vi "Read_Xml_Experiment.vi"(8 "error in":errorcluster) -> (0 "error out":errorcluster)   [LabVIEW 2023]
uses:
  TypeDef/Method_Info.ctl
panel:
  out "Method_Fit 2":T2
  in  "Method_Fit":T2
  in  "Method_Fit":T1[](array[typedef])
  out "Method_Fit":T1[](array[typedef])
  out "text":string
  in  "Xml path":path
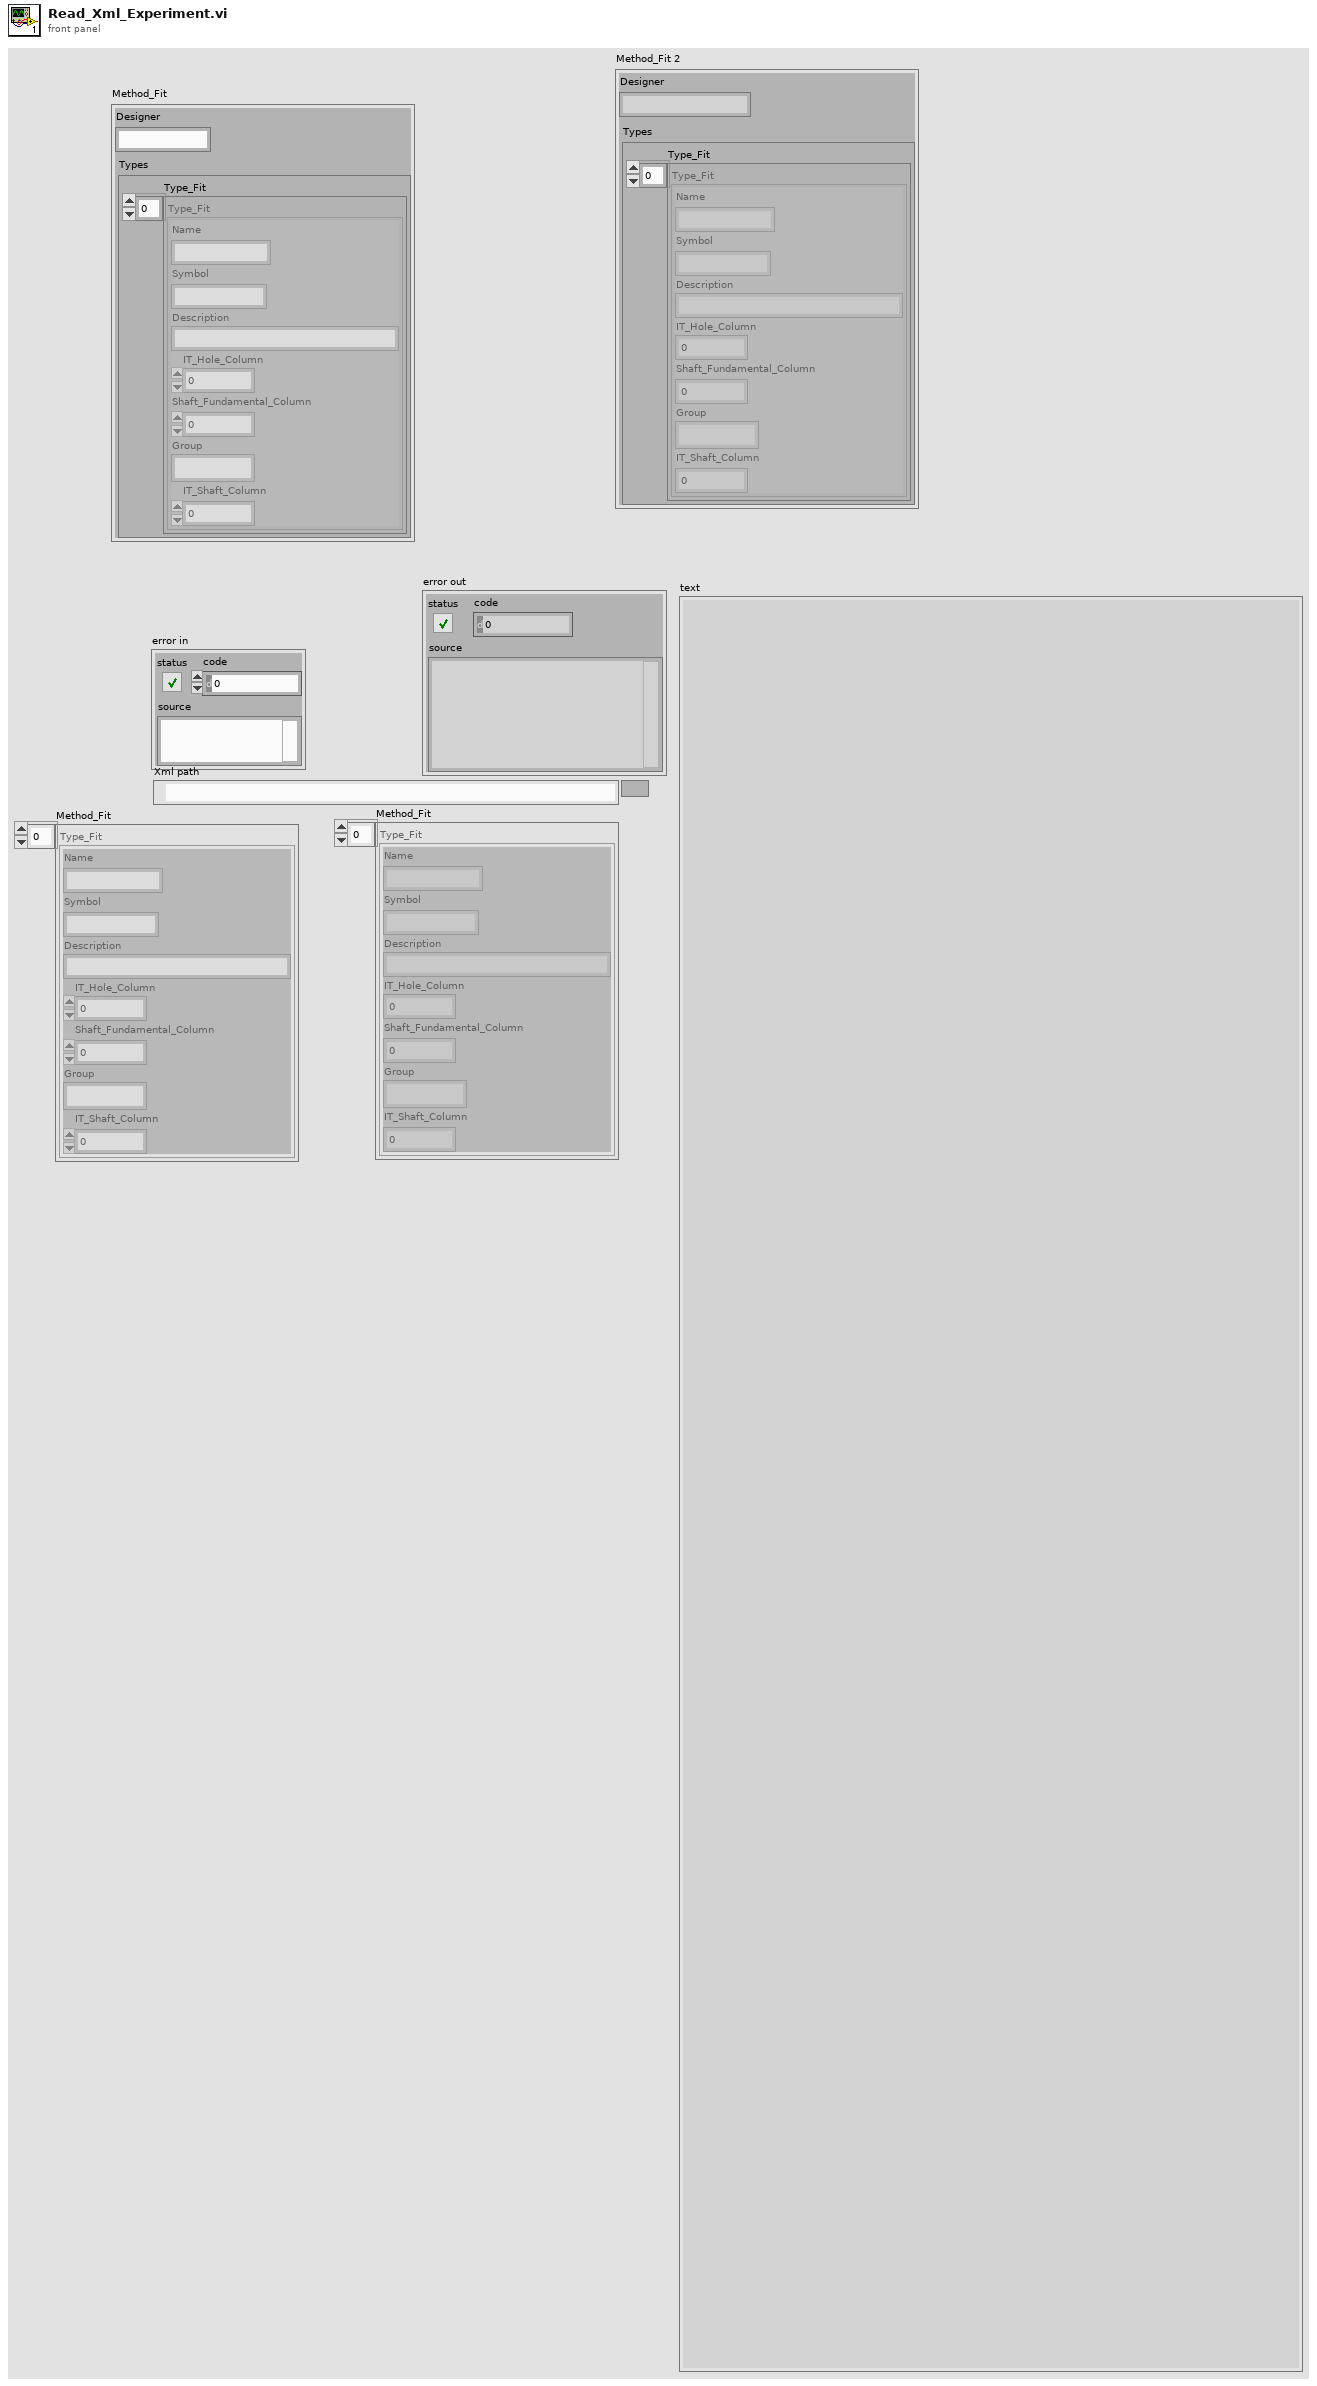
[diagram p1: front panel]
types:
  T1 = typedef "Method_Info.ctl" = cluster{"Name":string, "Symbol":string, "Description":string, "IT_Hole_Column":i32, "Shaft_Fundamental_Column":i32, "Group":string, "IT_Shaft_Column":i32}
  T2 = cluster{"Types":cluster{"Type_Fit":T1[]}, "Designer":string}
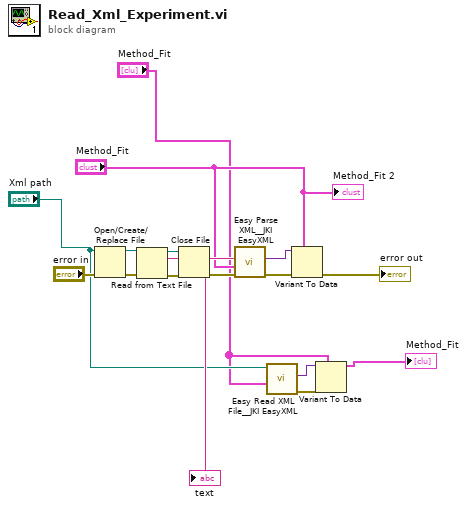
[diagram p0: block diagram]
diagram:
  n1 = Open/Create/Replace File(file path (use dialog)="Xml path", error in="error in") -> (refnum out=w13:refnum<file>, error out=w16:errorcluster)  [unwired: 4 in, 1 out]
  n2 = Read from Text File(file (use dialog)=w13, error in=w16) -> (refnum out=w14:refnum<file>, text=w9:string, error out=w15:errorcluster)  [unwired: 2 in, 1 out]
  "text" <- w9
  n3 = Close File(refnum=w14, error in=w15) -> (error out=w11:errorcluster)  [unwired: 1 out]
  n4 = call <vilib>:"Easy Parse XML__JKI EasyXML.vi"("error in (no error)"=w11, "LabVIEW Data (Type)"="Method_Fit", "XML String"=w9) -> ("error out"=w10:errorcluster, "LabVIEW Data"=w7:variant)  [unwired: 7 in]
  n5 = call <vilib>:"Easy Read XML File__JKI EasyXML.vi"("LabVIEW Data (Type)"="Method_Fit", "XML File Path"="Xml path") -> ("error out"=w5:errorcluster, "LabVIEW Data"=w4:variant)  [unwired: 7 in, 1 out]
  n6 = Variant To Data(error in=w10, type="Method_Fit", Variant=w7) -> (error out=→"error out":errorcluster)  [unwired: 1 out]
  n7 = Variant To Data(error in=w5, type="Method_Fit", Variant=w4) -> (data=→"Method_Fit":T1[])  [unwired: 1 out]
  "Method_Fit 2" <- "Method_Fit"
